vi "五参数标样核查.vi"(11 "启动参数":T1={"测量模式"=enum."标样核查", "数据标记表"="N", "输出参数"={"水温"=FALSE, "pH"=FALSE, "DO"=FALSE, "浊度"=FALSE, "电导率"=FALSE}}) -> ()   [LabVIEW 2016, in "斯坦道多参数.lvlib"]
panel:
  out "枚举":T2(ring)
  out "状态":string
  out "数值":i32
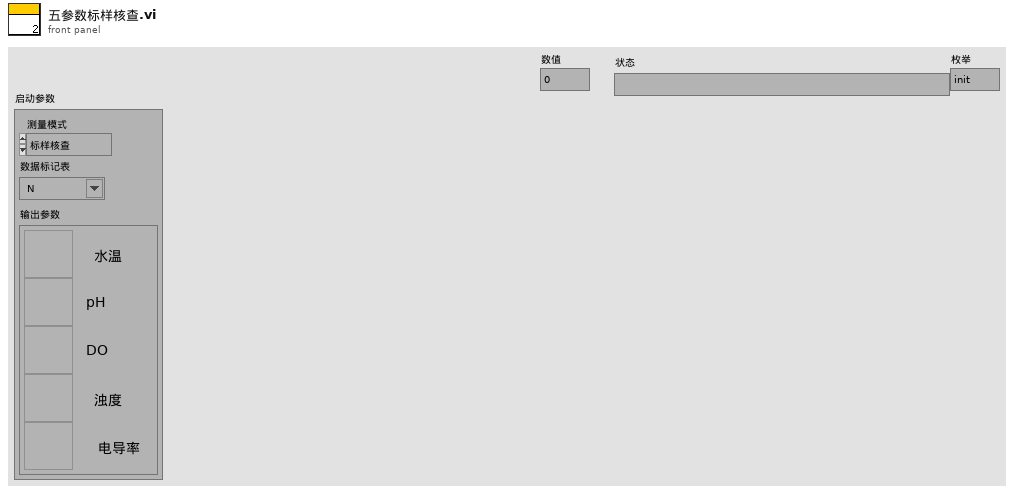
[diagram p1: front panel]
types:
  T1 = typedef "斯坦道多参数.lvlib/标样核查启动自定义输入参数.ctl" = cluster{"测量模式":enum16{"待机", "水样测试", "标样核查", "零点核查", "跨度核查", "空白测试", "平行样测试", "加标回收", "空白校准", "标样校准", "初始化（清洗）"}, "数据标记表":string, "输出参数":cluster{"水温":bool, "pH":bool, "DO":bool, "浊度":bool, "电导率":bool}}
  T2 = enum16{"init", "开机", "启动测量", "读取测量值", "存储数据", "关闭测量", "关机", "结束"}
  T3 = cluster{"时间标识":timestamp, "设备":string, "日志信息":string, "流程参数":string}
  T4 = cluster{"系统时间":timestamp, "工作状态":u16, "测量模式":u16, "告警代码":enum16{"无告警", "缺试剂告警", "缺水样告警", "缺蒸馏水告警", "缺标液告警", "仪表漏液告警", "标定异常告警", "超量程告警", "加热异常", "低试剂预警", "超上限告警", "超下限告警", "仪表内部其他异常", "滴定异常告警", "电极异常告警", "量程切换告警", "参数设置告警", "PH电极电位异常", "电导率电极异常", "浊度光度异常", "溶解氧电极异常", "溶解氧光强异常", "温度异常告警", "PH异常告警", "溶解氧异常告警", "电导率异常告警", "浊度异常告警", "叶绿素异常告警", "藻密度异常告警", "蓝绿藻异常告警", "ORP异常告警", "氨氮异常告警", "清洁刷异常告警", "SD卡异常告警", "蓝牙异常告警", "Wifi异常告警", "流程异常告警"}, "故障代码":enum16{"无故障", "电机故障", "温度故障", "通讯故障", "滴定故障"}, "日志代码":u16, "软件版本":string}
  T5 = enum16{"待机", "水样测试", "标样核查", "零点核查", "跨度核查", "空白测试", "平行样测试", "加标回收", "空白校准", "标样校准", "初始化（清洗）"}
  T6 = cluster{"数据标记表":string, "测量模式":enum16{"待机", "水样测试", "标样核查", "零点核查", "跨度核查", "空白测试", "平行样测试", "加标回收", "空白校准", "标样校准", "初始化（清洗）"}}
  T7 = cluster{"水温标准液标准浓度":dbl, "酸碱度标准液标准浓度":dbl, "溶解氧标准液标准浓度":dbl, "电导率标准液标准浓度":dbl, "浊度标准液标准浓度":dbl}
  T8 = cluster{"因子编码":string, "单位":string, "标样参考值":sgl, "水样数据时间":timestamp, "水样实测值":sgl, "水样数据标识":string, "K":sgl, "B":sgl, "T":sgl, "H":sgl, "水深":sgl, "探头温度":sgl}
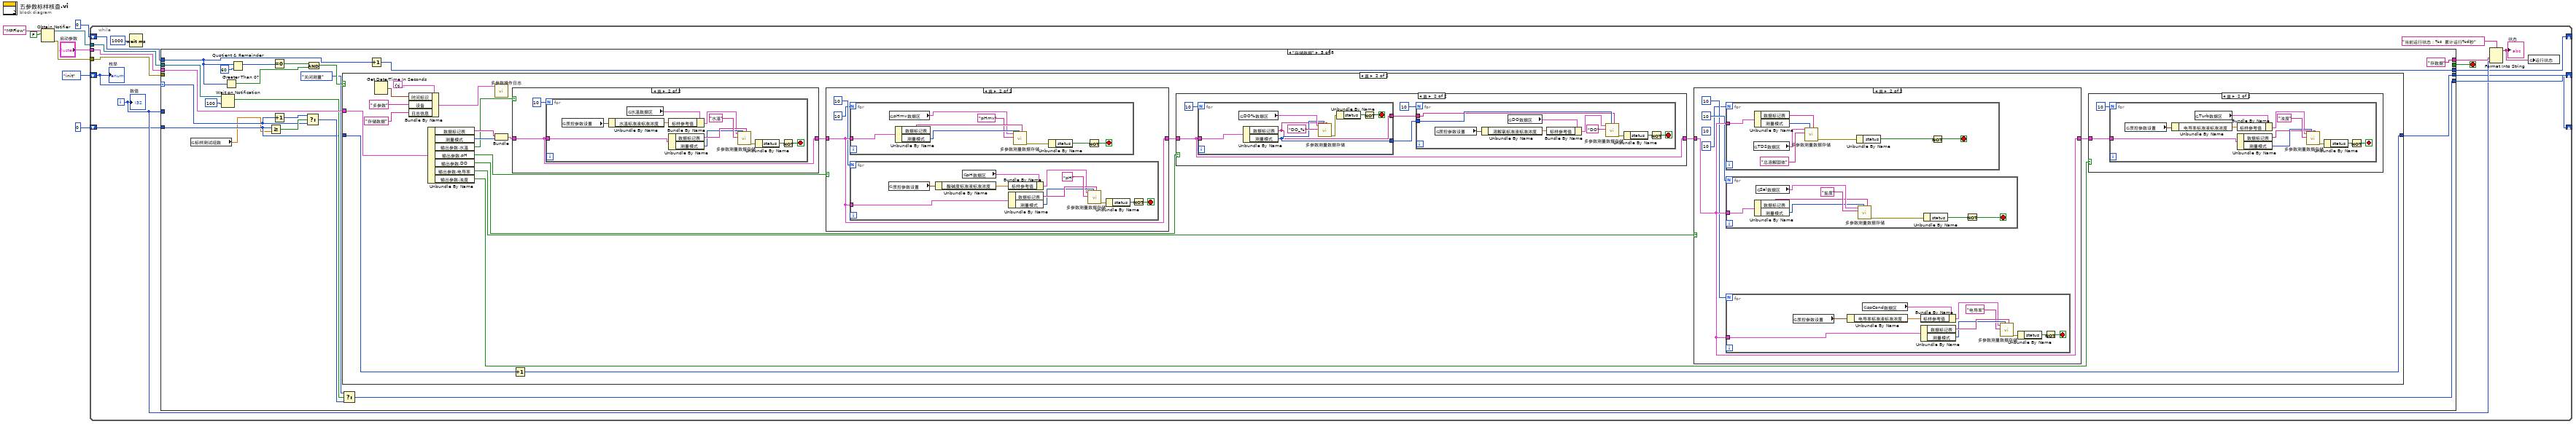
[diagram p0: block diagram]
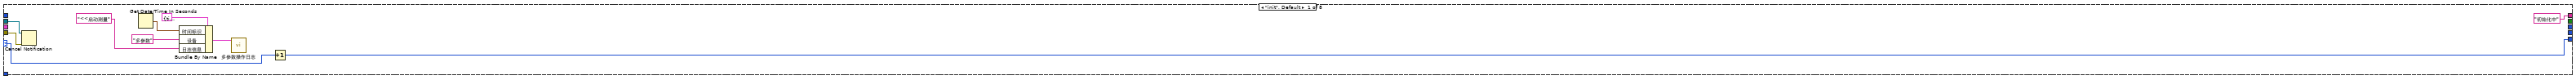
[diagram p2: hidden frame]
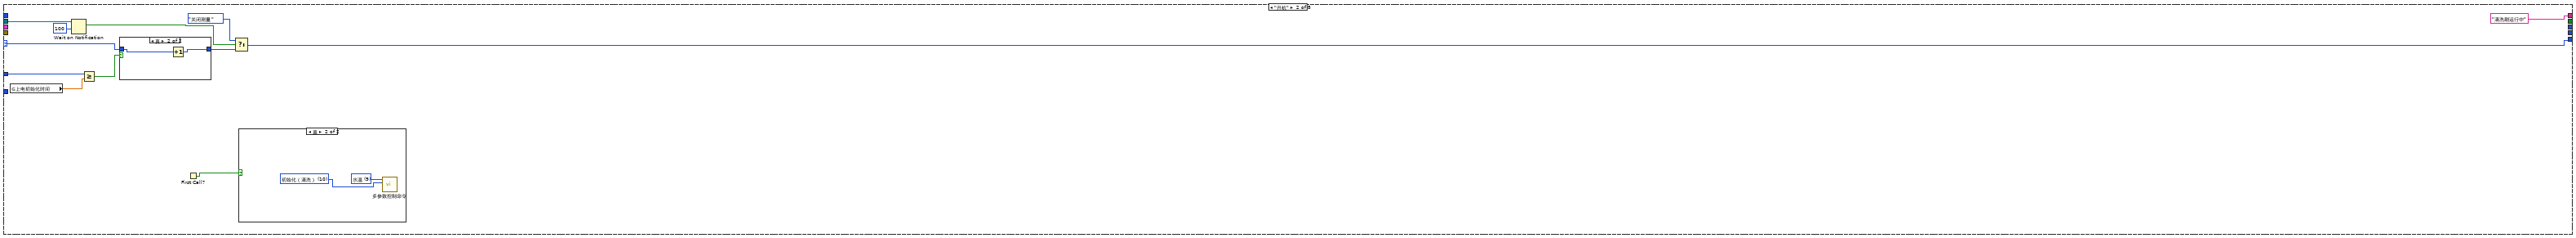
[diagram p3: hidden frame]
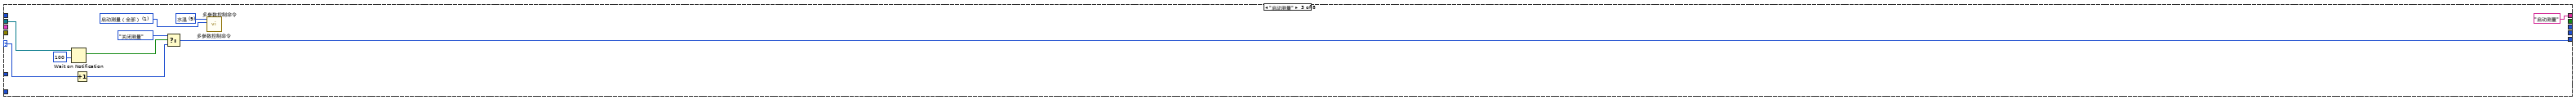
[diagram p6: hidden frame]
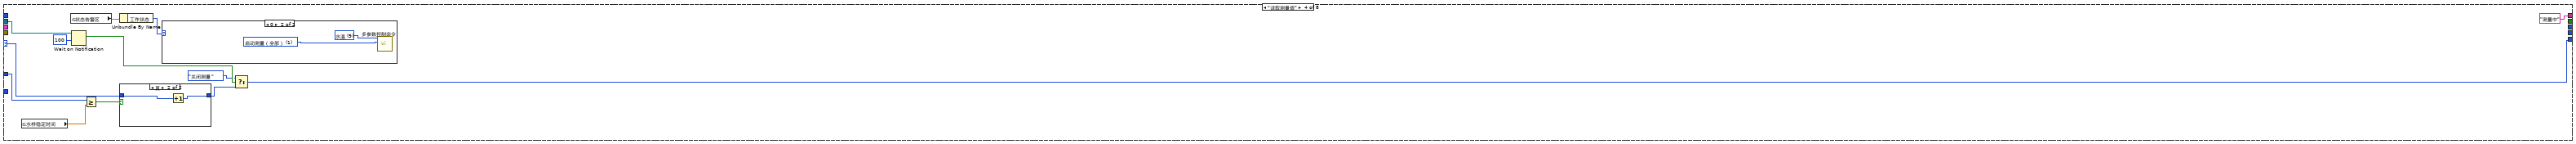
[diagram p7: hidden frame]
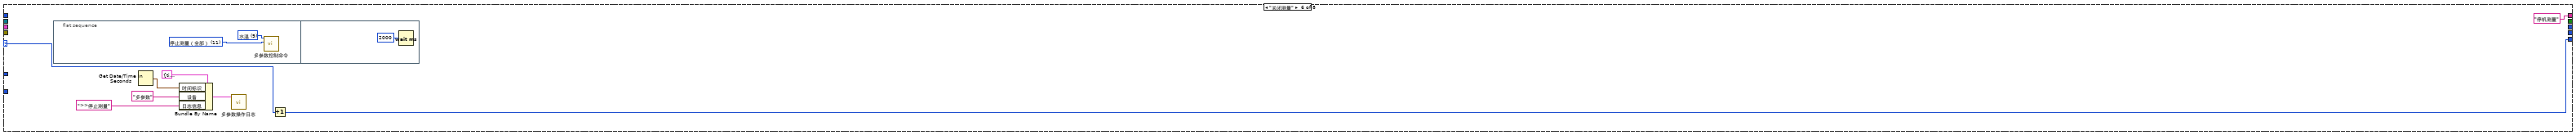
[diagram p16: hidden frame]
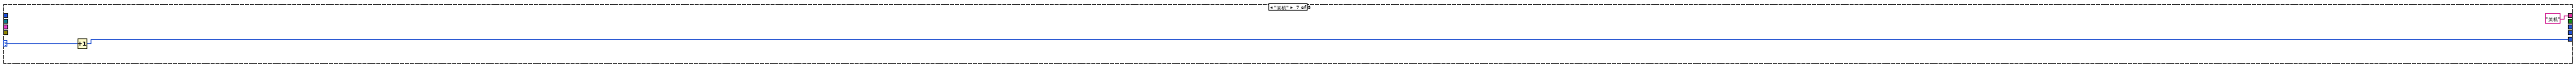
[diagram p17: hidden frame]
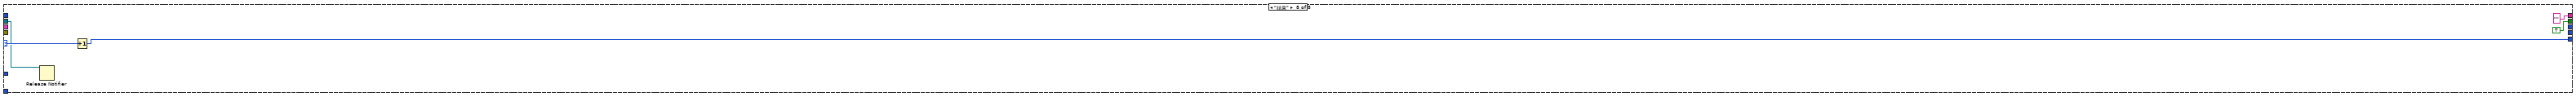
[diagram p18: hidden frame]
diagram:
  n1 = Obtain Notifier(name (unnamed)="MPFlow" ("名称（未命名）"), notification data type=FALSE) -> (notifier out=w5:refnum<notifier>, error out=w4:errorcluster)  [unwired: 2 in, 1 out]
  n2 = while {
    shift-right: [w19] -> _
    shift-left: T2."init" ("枚举") -> [w23]
    tunnel: w5 -> [w21]
    tunnel: w4 -> [w20]
    tunnel: "启动参数" -> [w13]
    shift-right: [w11] -> _
    shift-left: u32 0 ("等待时间（毫秒）") -> [w12]
    shift-right: [w9] -> _
    shift-left: u32 0 ("等待时间（毫秒）") -> [w10]
    i -> [w15]
    stop <- w22 stop-if-true
    n3 = Wait (ms)(milliseconds to wait=u32 1000 ("等待时间（毫秒）")) -> ()  [unwired: 1 out]
    n4 = case shown="\"存储数据\"" w23 {
      selector: w23 -> [w31 w45 w62 w75 w82 w236 w242 w246]
      tunnel: [_ _ _ _ _ _ _ TRUE] -> w22
      tunnel: w21 -> [w33 w41 w61 w72 w91 _ _ w243]
      tunnel: w20 -> [w32 _ _ _ _ _ _ _]
      tunnel: [w30 w39 w58 w70 w87 w235 w241 w245] -> w19
      tunnel: w15 -> [_ w44 _ w66 _ _ _ _]
      tunnel: ["初始化中" ("状态") "清洗刷运行中" ("状态") "启动测量" ("状态") "测量中" ("状态") "存数据" ("状态") "停机测量" ("状态") "关机" ("状态") "" ("状态")] -> w16
      tunnel: w13 -> [_ _ _ _ w100 _ _ _]
      tunnel: w12 -> [_ _ _ _ w94 _ _ _]
      tunnel: [_ _ _ _ w95 _ _ _] -> w11
      tunnel: w10 -> [_ _ _ _ w84 _ _ _]
      tunnel: [_ _ _ _ w86 _ _ _] -> w9
      frame "init", Default {
        n5 = Cancel Notification(0:w33, 3:w32) -> ()  [unwired: 3 out]
        n6 = Get Date/Time In Seconds() -> (seconds since 1Jan1904=w27:timestamp)
        n7 = Bundle By Name(cluster=T3 {"时间标识"=timestamp(0 s since 1904-01-01), "设备"="", "日志信息"="", "流程参数"=""} ("data in"), "时间标识"=w27, "设备"="多参数", "日志信息"="<<启动测量") -> (w26:T3)
        n8 = call "多参数操作日志.vi"("data in"=w26) -> ()  [unwired: 10 in, 1 out]
        n9 = Increment(x=w31) -> (x+1=w30:T2)
      }
      frame "开机" {
        n10 = global read "多参数断电保存全局变量.vi" "上电初始化时间"() -> (w34:dbl)
        n11 = Wait on Notification(notifier=w41, timeout in ms (-1)=100 ("超时毫秒(-1)")) -> (notification=w42:bool)  [unwired: 2 in, 3 out]
        n12 = Greater Or Equal?(x=w44, y=w34) -> (x >= y?=w43:bool)
        n13 = case shown="真" w43 {
          tunnel: w45 -> [w48 w50]
          tunnel: [w48 w49] -> w40
          frame False {
          }
          frame True {
            n14 = Increment(x=w50) -> (x+1=w49:T2)
          }
        }
        n15 = First Call?() -> (First Call?: T/F=w35:bool)
        n16 = Select(t=T2."关闭测量" ("枚举"), s=w42, f=w40) -> (s? t:f=w39:T2)
        n17 = case shown="真" w35 {
          frame False {
          }
          frame True {
            w47 = u16 10 items=["启动测量（全部）"=1, "初始化（清洗）"=10, "停止测量（全部）"=11, "校时"=13, "启动测量（单个传感器）"=19, "停止测量（单个传感器）"=20] ("控制命令")
            w46 = u16 9 items=["氨氮"=3, "水温"=9, "pH值"=10, "溶解氧"=11, "电导率"=12, "浊度"=13, "叶绿素a"=14, "藻密度"=15, "蓝绿藻"=16, "氧化还原电位"=17, "溶解氧%"=18, "盐度"=19] ("站号")
            n18 = call "多参数控制命令.vi"("控制命令"=w47, "站号"=w46) -> ()  [unwired: 9 in, 1 out]
          }
        }
      }
      frame "启动测量" {
        w52 = u16 1 items=["启动测量（全部）"=1, "初始化（清洗）"=10, "停止测量（全部）"=11, "校时"=13, "启动测量（单个传感器）"=19, "停止测量（单个传感器）"=20] ("控制命令")
        w51 = u16 9 items=["氨氮"=3, "水温"=9, "pH值"=10, "溶解氧"=11, "电导率"=12, "浊度"=13, "叶绿素a"=14, "藻密度"=15, "蓝绿藻"=16, "氧化还原电位"=17, "溶解氧%"=18, "盐度"=19] ("站号")
        w53 = u16 1 items=["启动测量（全部）"=1, "初始化（清洗）"=10, "停止测量（全部）"=11, "校时"=13, "启动测量（单个传感器）"=19, "停止测量（单个传感器）"=20] ("控制命令")
        w54 = u16 9 items=["氨氮"=3, "水温"=9, "pH值"=10, "溶解氧"=11, "电导率"=12, "浊度"=13, "叶绿素a"=14, "藻密度"=15, "蓝绿藻"=16, "氧化还原电位"=17, "溶解氧%"=18, "盐度"=19] ("站号")
        n19 = Wait on Notification(notifier=w61, timeout in ms (-1)=100 ("超时毫秒(-1)")) -> (notification=w60:bool)  [unwired: 2 in, 3 out]
        n20 = Increment(x=w62) -> (x+1=w59:T2)
        n21 = Select(t=T2."关闭测量" ("枚举"), s=w60, f=w59) -> (s? t:f=w58:T2)
        n22 = call "多参数控制命令.vi"("控制命令"=w52, "站号"=w51) -> ()  [unwired: 9 in, 1 out]
        n23 = call "多参数控制命令.vi"("控制命令"=w53, "站号"=w54) -> ()  [unwired: 9 in, 1 out]
      }
      frame "读取测量值" {
        n24 = global read "多参数断电保存全局变量.vi" "水样稳定时间"() -> (w63:dbl)
        n25 = global read "多参数全局变量.vi" "状态告警区"() -> (w65:T4)
        n26 = Wait on Notification(notifier=w72, timeout in ms (-1)=100 ("超时毫秒(-1)")) -> (notification=w73:bool)  [unwired: 2 in, 3 out]
        n27 = Greater Or Equal?(x=w66, y=w63) -> (x >= y?=w74:bool)
        n28 = Unbundle By Name(w65) -> ("工作状态"=w64:u16)
        n29 = case shown="真" w74 {
          tunnel: w75 -> [w78 w80]
          tunnel: [w78 w79] -> w71
          frame False {
          }
          frame True {
            n30 = Increment(x=w80) -> (x+1=w79:T2)
          }
        }
        n31 = case shown="0" w64 {
          frame Default {
          }
          frame 0 {
            w76 = u16 1 items=["启动测量（全部）"=1, "初始化（清洗）"=10, "停止测量（全部）"=11, "校时"=13, "启动测量（单个传感器）"=19, "停止测量（单个传感器）"=20] ("控制命令")
            w77 = u16 9 items=["氨氮"=3, "水温"=9, "pH值"=10, "溶解氧"=11, "电导率"=12, "浊度"=13, "叶绿素a"=14, "藻密度"=15, "蓝绿藻"=16, "氧化还原电位"=17, "溶解氧%"=18, "盐度"=19] ("站号")
            n32 = call "多参数控制命令.vi"("控制命令"=w76, "站号"=w77) -> ()  [unwired: 9 in, 1 out]
          }
        }
        n33 = Select(t=T2."关闭测量" ("枚举"), s=w73, f=w71) -> (s? t:f=w70:T2)
      }
      frame "存储数据" {
        n34 = global read "多参数断电保存全局变量.vi" "标样测试组数"() -> (w81:dbl)
        n35 = Wait on Notification(notifier=w91, timeout in ms (-1)=100 ("超时毫秒(-1)")) -> (notification=w90:bool)  [unwired: 2 in, 3 out]
        n36 = Greater Than 0?(x=w94) -> (x > 0?=w93:bool)
        n37 = Quotient & Remainder(x=w94, y=u32 60) -> (x-y*floor(x/y)=w98:u32)  [unwired: 1 out]
        n38 = Greater Or Equal?(x=w84, y=w81) -> (x >= y?=w85:bool)
        n39 = Equal To 0?(x=w98) -> (x = 0?=w97:bool)
        n40 = Increment(x=w82) -> (x+1=w83:T2)
        n41 = Select(t=w83, s=w85, f=w82) -> (s? t:f=w89:T2)
        n42 = Compound Arithmetic op=AND ("复合运算")(w97, w93) -> (w96:bool)
        n43 = case shown="真" w96 {
          tunnel: w100 -> [_ w122]
          tunnel: w84 -> [w102 w104]
          tunnel: [w102 w103] -> w86
          frame False {
          }
          frame True {
            n44 = Get Date/Time In Seconds() -> (seconds since 1Jan1904=w113:timestamp)
            n45 = Bundle By Name(cluster=T3 {"时间标识"=timestamp(0 s since 1904-01-01), "设备"="", "日志信息"="", "流程参数"=""} ("data in"), "时间标识"=w113, "设备"="多参数", "日志信息"="存储数据") -> (w112:T3)
            n46 = Unbundle By Name(w122) -> ("数据标记表"=w121:string, "测量模式"=w120:T5, "输出参数.水温"=w109:bool, "输出参数.pH"=w108:bool, "输出参数.DO"=w107:bool, "输出参数.电导率"=w106:bool, "输出参数.浊度"=w105:bool)
            n47 = call "多参数操作日志.vi"("data in"=w112) -> ()  [unwired: 10 in, 1 out]
            n48 = Bundle("数据标记表"=w121, "测量模式"=w120) -> (w119:T6)  [unwired: 1 in]
            n49 = case shown="真" w109 {
              tunnel: w119 -> [w215 w217]
              tunnel: [w215 w217] -> w118
              frame False {
              }
              frame True {
                n50 = for {
                  N: 10 -> [_]
                  tunnel: w217 -> [w227]
                  stop <- w218 stop-if-true
                  n51 = global read "多参数断电保存全局变量.vi" "质控参数设置"() -> (w223:T7)
                  n52 = Unbundle By Name(w223) -> ("水温标准液标准浓度"=w222:dbl)
                  n53 = global read "多参数全局变量.vi" "水温数据区"() -> (w224:T8)
                  n54 = Bundle By Name(cluster=w224, "标样参考值"=w222) -> (w221:T8)
                  n55 = Unbundle By Name(w227) -> ("数据标记表"=w226:string, "测量模式"=w225:T5)
                  n56 = call "多参数测量数据存储.vi"("数据类型"=w226, "测量模式"=w225, "table输入"="水温", "data in"=w221) -> ("error out"=w220:errorcluster)  [unwired: 7 in]
                  n57 = Unbundle By Name(w220) -> ("status"=w219:bool)
                  n58 = Not(x=w219) -> (.not. x?=w218:bool)
                }
              }
            }
            n59 = Increment(x=w104) -> (x+1=w103:u32)
            n60 = case shown="真" w108 {
              tunnel: w118 -> [w192 w195]
              tunnel: [w192 w195] -> w116
              frame False {
              }
              frame True {
                n61 = for {
                  N: 10 -> [_]
                  tunnel: w195 -> [w203]
                  stop <- w196 stop-if-true
                  n62 = global read "多参数全局变量.vi" "pHmv数据区"() -> (w200:T8)
                  n63 = Unbundle By Name(w203) -> ("数据标记表"=w202:string, "测量模式"=w201:T5)
                  n64 = call "多参数测量数据存储.vi"("数据类型"=w202, "测量模式"=w201, "table输入"="pHmv", "data in"=w200) -> ("error out"=w198:errorcluster)  [unwired: 7 in]
                  n65 = Unbundle By Name(w198) -> ("status"=w197:bool)
                  n66 = Not(x=w197) -> (.not. x?=w196:bool)
                }
                n67 = for {
                  N: 10 -> [_]
                  tunnel: w195 -> [w211]
                  stop <- w204 stop-if-true
                  n68 = global read "多参数断电保存全局变量.vi" "质控参数设置"() -> (w210:T7)
                  n69 = Unbundle By Name(w210) -> ("酸碱度标准液标准浓度"=w209:dbl)
                  n70 = global read "多参数全局变量.vi" "pH数据区"() -> (w208:T8)
                  n71 = Bundle By Name(cluster=w208, "标样参考值"=w209) -> (w207:T8)
                  n72 = Unbundle By Name(w211) -> ("数据标记表"=w213:string, "测量模式"=w212:T5)
                  n73 = call "多参数测量数据存储.vi"("数据类型"=w213, "测量模式"=w212, "table输入"="pH", "data in"=w207) -> ("error out"=w206:errorcluster)  [unwired: 7 in]
                  n74 = Unbundle By Name(w206) -> ("status"=w205:bool)
                  n75 = Not(x=w205) -> (.not. x?=w204:bool)
                }
              }
            }
            n76 = case shown="真" w107 {
              tunnel: [w168 w173] -> w117
              tunnel: w116 -> [w168 w173]
              frame False {
              }
              frame True {
                n77 = for {
                  N: 10 -> [_]
                  tunnel: w173 -> [w189]
                  tunnel: [w188] -> w172
                  tunnel: [w187] -> w171
                  stop <- w184 stop-if-true
                  n78 = global read "多参数全局变量.vi" "DO%数据区"() -> (w191:T8)
                  n79 = Unbundle By Name(w189) -> ("数据标记表"=w187:string, "测量模式"=w188:T5)
                  n80 = call "多参数测量数据存储.vi"("数据类型"=w187, "测量模式"=w188, "table输入"="DO_%", "data in"=w191) -> ("error out"=w186:errorcluster)  [unwired: 7 in]
                  n81 = Unbundle By Name(w186) -> ("status"=w185:bool)
                  n82 = Not(x=w185) -> (.not. x?=w184:bool)
                }
                n83 = for {
                  N: 10 -> [_]
                  tunnel: w172 -> [w182]
                  tunnel: w171 -> [w181]
                  stop <- w174 stop-if-true
                  n84 = global read "多参数断电保存全局变量.vi" "质控参数设置"() -> (w180:T7)
                  n85 = Unbundle By Name(w180) -> ("溶解氧标准液标准浓度"=w179:dbl)
                  n86 = global read "多参数全局变量.vi" "DO数据区"() -> (w178:T8)
                  n87 = Bundle By Name(cluster=w178, "标样参考值"=w179) -> (w177:T8)
                  n88 = call "多参数测量数据存储.vi"("数据类型"=w181, "测量模式"=w182, "table输入"="DO", "data in"=w177) -> ("error out"=w176:errorcluster)  [unwired: 7 in]
                  n89 = Unbundle By Name(w176) -> ("status"=w175:bool)
                  n90 = Not(x=w175) -> (.not. x?=w174:bool)
                }
              }
            }
            n91 = case shown="真" w106 {
              tunnel: w117 -> [w136 w140]
              tunnel: [w136 w140] -> w115
              frame False {
              }
              frame True {
                (unwired) 10
                n92 = for {
                  N: 10 -> [_]
                  tunnel: w140 -> [w148]
                  stop <- w141 stop-if-true
                  n93 = global read "多参数全局变量.vi" "TDS数据区"() -> (w145:T8)
                  n94 = Unbundle By Name(w148) -> ("数据标记表"=w146:string, "测量模式"=w147:T5)
                  n95 = call "多参数测量数据存储.vi"("数据类型"=w146, "测量模式"=w147, "table输入"="总溶解固体", "data in"=w145) -> ("error out"=w143:errorcluster)  [unwired: 7 in]
                  n96 = Unbundle By Name(w143) -> ("status"=w142:bool)
                  n97 = Not(x=w142) -> (.not. x?=w141:bool)
                }
                n98 = for {
                  N: 10 -> [_]
                  tunnel: w140 -> [w163]
                  stop <- w160 stop-if-true
                  n99 = Unbundle By Name(w163) -> ("数据标记表"=w165:string, "测量模式"=w164:T5)
                  n100 = global read "多参数全局变量.vi" "Sal数据区"() -> (w167:T8)
                  n101 = call "多参数测量数据存储.vi"("数据类型"=w165, "测量模式"=w164, "table输入"="盐度", "data in"=w167) -> ("error out"=w162:errorcluster)  [unwired: 7 in]
                  n102 = Unbundle By Name(w162) -> ("status"=w161:bool)
                  n103 = Not(x=w161) -> (.not. x?=w160:bool)
                }
                n104 = for {
                  N: 10 -> [_]
                  tunnel: w140 -> [w159]
                  stop <- w149 stop-if-true
                  n105 = global read "多参数断电保存全局变量.vi" "质控参数设置"() -> (w155:T7)
                  n106 = Unbundle By Name(w155) -> ("电导率标准液标准浓度"=w154:dbl)
                  n107 = global read "多参数全局变量.vi" "spCond数据区"() -> (w153:T8)
                  n108 = Bundle By Name(cluster=w153, "标样参考值"=w154) -> (w152:T8)
                  n109 = Unbundle By Name(w159) -> ("数据标记表"=w158:string, "测量模式"=w157:T5)
                  n110 = call "多参数测量数据存储.vi"("数据类型"=w158, "测量模式"=w157, "table输入"="电导率", "data in"=w152) -> ("error out"=w151:errorcluster)  [unwired: 7 in]
                  n111 = Unbundle By Name(w151) -> ("status"=w150:bool)
                  n112 = Not(x=w150) -> (.not. x?=w149:bool)
                }
              }
            }
            n113 = case shown="真" w105 {
              tunnel: w115 -> [_ w124]
              frame False {
              }
              frame True {
                n114 = for {
                  N: 10 -> [_]
                  tunnel: w124 -> [w134]
                  stop <- w125 stop-if-true
                  n115 = global read "多参数断电保存全局变量.vi" "质控参数设置"() -> (w131:T7)
                  n116 = Unbundle By Name(w131) -> ("电导率标准液标准浓度"=w130:dbl)
                  n117 = global read "多参数全局变量.vi" "Turb数据区"() -> (w129:T8)
                  n118 = Bundle By Name(cluster=w129, "标样参考值"=w130) -> (w128:T8)
                  n119 = Unbundle By Name(w134) -> ("数据标记表"=w132:string, "测量模式"=w133:T5)
                  n120 = call "多参数测量数据存储.vi"("数据类型"=w132, "测量模式"=w133, "table输入"="浊度", "data in"=w128) -> ("error out"=w127:errorcluster)  [unwired: 7 in]
                  n121 = Unbundle By Name(w127) -> ("status"=w126:bool)
                  n122 = Not(x=w126) -> (.not. x?=w125:bool)
                }
              }
            }
          }
        }
        n123 = Select(t=T2."关闭测量", s=w90, f=w89) -> (s? t:f=w87:T2)
        n124 = Increment(x=w94) -> (x+1=w95:u32)
      }
      frame "关闭测量" {
        n125 = flat-sequence {
          frame #0 {
            w237 = u16 11 items=["启动测量（全部）"=1, "初始化（清洗）"=10, "停止测量（全部）"=11, "校时"=13, "启动测量（单个传感器）"=19, "停止测量（单个传感器）"=20] ("控制命令")
            w238 = u16 9 items=["氨氮"=3, "水温"=9, "pH值"=10, "溶解氧"=11, "电导率"=12, "浊度"=13, "叶绿素a"=14, "藻密度"=15, "蓝绿藻"=16, "氧化还原电位"=17, "溶解氧%"=18, "盐度"=19] ("站号")
            n126 = call "多参数控制命令.vi"("控制命令"=w237, "站号"=w238) -> ()  [unwired: 9 in, 1 out]
          }
          frame #1 {
            n127 = Wait (ms)(milliseconds to wait=u32 2000 ("等待时间（毫秒）")) -> ()  [unwired: 1 out]
          }
        }
        n128 = Get Date/Time In Seconds() -> (seconds since 1Jan1904=w232:timestamp)
        n129 = Bundle By Name(cluster=T3 {"时间标识"=timestamp(0 s since 1904-01-01), "设备"="", "日志信息"="", "流程参数"=""} ("data in"), "时间标识"=w232, "设备"="多参数", "日志信息"=">>停止测量") -> (w231:T3)
        n130 = call "多参数操作日志.vi"("data in"=w231) -> ()  [unwired: 10 in, 1 out]
        n131 = Increment(x=w236) -> (x+1=w235:T2)
      }
      frame "关机" {
        n132 = Increment(x=w242) -> (x+1=w241:T2)
      }
      frame "结束" {
        n133 = Release Notifier(notifier=w243) -> ()  [unwired: 2 in, 3 out]
        n134 = Increment(x=w246) -> (x+1=w245:T2)
      }
    }
    n135 = Format Into String(format string="当前运行状态：%s  累计运行%d秒" ("格式字符串"), w16, w15) -> (resulting string=w14:string)  [unwired: 2 in, 1 out]
    "状态" <- w14
    n136 = global write "多参数全局变量.vi" "运行状态"(w14) -> ()
    "数值" <- w15
    "枚举" <- w23
  }
